vi "Create Data Frame FCS.vi"(0 "Data":u8=128, 1 "OVS":u8=16, 5 "Num_of_FCS_Bits":u8=4, 7 "Polynomial_Mask":u8=19 format="%.0x", 11 "error in (no error)":errorcluster, 12 "sample rate":dbl=1000.0 format="%#_6p") -> (4 "Digital Waveform Graph_Out":digitalwaveform(graph), 15 "error out":errorcluster)   [LabVIEW 2013]
panel:
  out "Final_DATA_Frame":bool[](array[boolean])
  out "All_Decoding_Steps":bool[][](array[boolean])
  out "FCS_Value":u32
  out "Final_Data_FCS":bool[](array[boolean])
  out "Data_FCS":bool[](array[boolean])
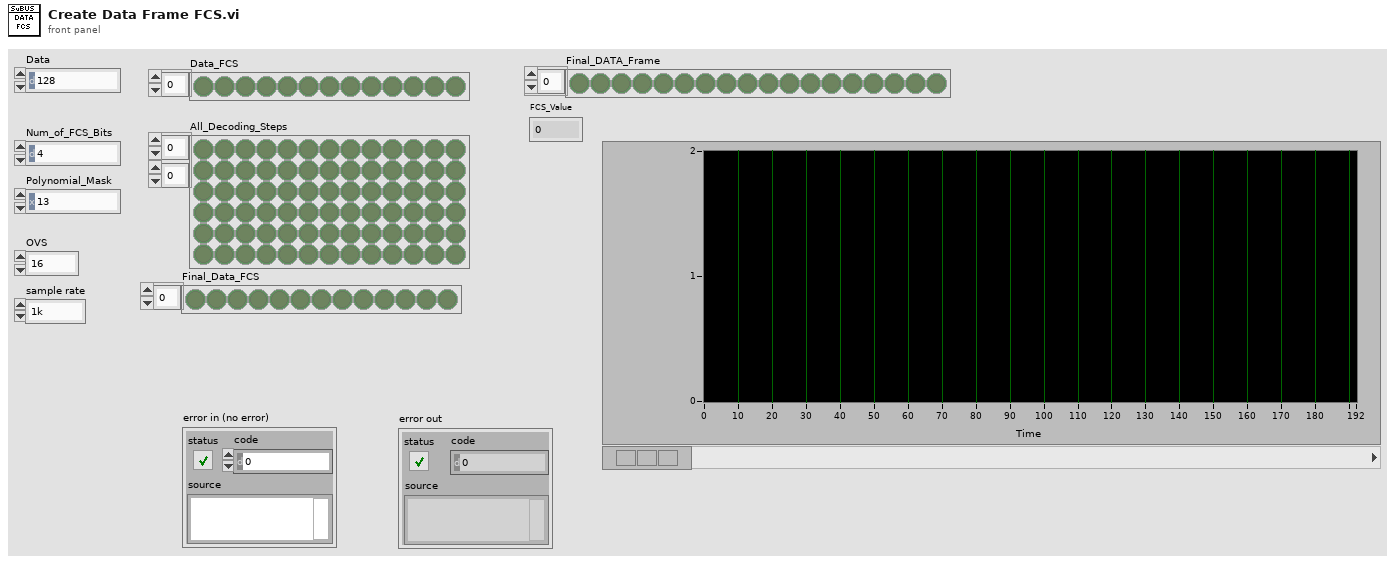
[diagram p1: front panel]
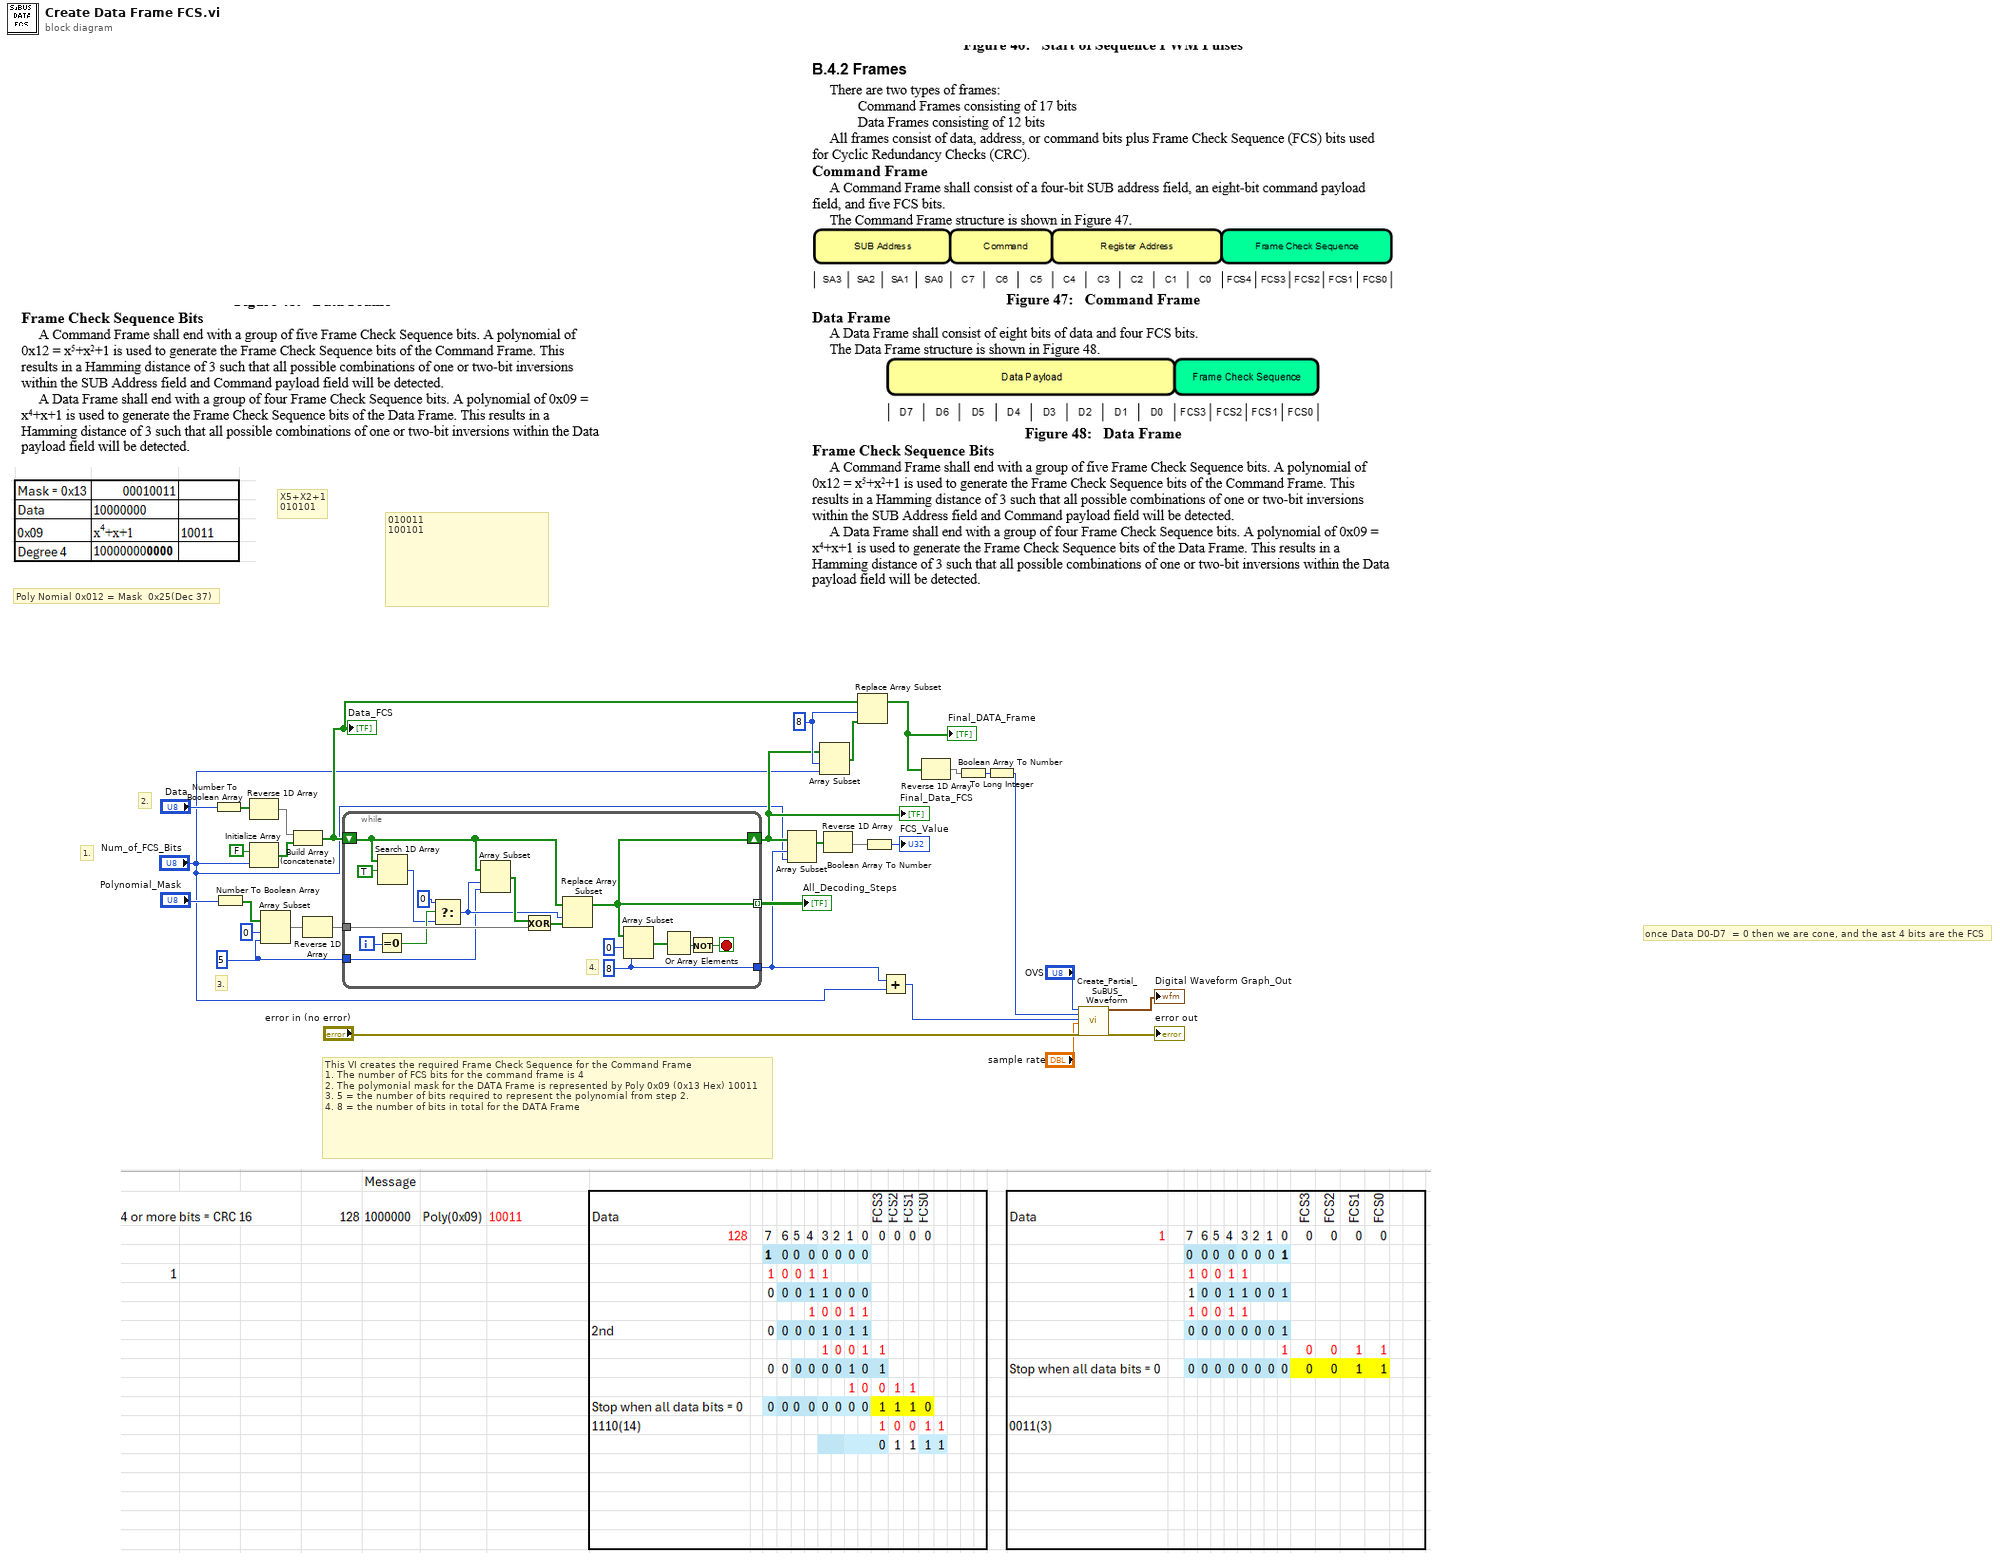
[diagram p0: block diagram]
diagram:
  w6 = 8 ("index")
  w18 = 5 ("length")
  # "3."
  # "2."
  # "1."
  # "This VI creates the required Frame Check Sequence for the Command Frame\n1. The number of FCS bits for the command frame is 4 \n2. The polymonial mask for the DATA Frame is represented by Poly 0x09 (0x13 Hex) 10011\n3. 5 = the number of bits required to represent the polynomial from step 2.\n4. 8 = the number of bits in total for the DATA Frame"
  # "Poly Nomial 0x012 = Mask  0x25(Dec 37)"
  # "010011\n100101"
  # "X5+X2+1\n010101"
  # "once Data D0-D7  = 0 then we are cone, and the ast 4 bits are the FCS"
  n1 = Number To Boolean Array(number="Data") -> (Boolean array=w28:bool[])
  n2 = Number To Boolean Array(number="Polynomial_Mask") -> (Boolean array=w31:bool[])
  n3 = Reverse 1D Array(array=w28) -> (reversed array=w26:bool[])
  n4 = Initialize Array(FALSE ("element"), "Num_of_FCS_Bits") -> (w25:bool[])
  n5 = Array Subset(array=w31, index=0, length=w18) -> (w30:bool[])
  n6 = Build Array (concatenate)(w26, w25) -> (w5:bool[])
  "Data_FCS" <- w5
  n7 = Reverse 1D Array(array=w30) -> (reversed array=w24:bool[])
  n8 = while {
    shift-right: [w34] -> w4
    shift-left: w5 -> [w41]
    tunnel: w24 -> [w48]
    tunnel: [w34] -> w21 mode=indexing
    tunnel: w18 -> [w33]
    tunnel: [w32] -> w10
    i -> [w39]
    stop <- w42 stop-if-true
    w32 = 8 ("length")
    # "4."
    n9 = Equal To 0?(x=w39) -> (x = 0?=w38:bool)
    n10 = Search 1D Array(1D array=w41, element=TRUE) -> (index of element=w37:i32)  [unwired: 1 in]
    n11 = Select(t=0, s=w38, f=w37) -> (s? t:f=w36:i32)
    n12 = Array Subset(array=w41, index=w36, length=w33) -> (w47:bool[])
    n13 = Exclusive Or(1:w48, 2:w47) -> (0:w40:bool[])
    n14 = Replace Array Subset(array=w41, new element=w40, index=w36) -> (w34:bool[])
    n15 = Array Subset(array=w34, index=0, length=w32) -> (w45:bool[])
    n16 = Or Array Elements(Boolean array=w45) -> (logical OR=w44:bool)
    n17 = Not(x=w44) -> (.not. x?=w42:bool)
  }
  "Final_Data_FCS" <- w4
  "All_Decoding_Steps" <- w21
  n18 = Array Subset(array=w4, index=w10, length="Num_of_FCS_Bits") -> (w22:bool[])
  n19 = Array Subset(array=w4, index=w6, length="Num_of_FCS_Bits") -> (w7:bool[])
  n20 = Reverse 1D Array(array=w22) -> (reversed array=w17:bool[])
  n21 = Replace Array Subset(array=w5, new element=w7, index=w6) -> (w1:bool[])
  "Final_DATA_Frame" <- w1
  n22 = Boolean Array To Number(Boolean array=w17) -> (number=→"FCS_Value":u32)
  n23 = Add(x=w10, y="Num_of_FCS_Bits") -> (x+y=w9:i32)
  n24 = Reverse 1D Array(array=w1) -> (reversed array=w2:bool[])
  n25 = Boolean Array To Number(Boolean array=w2) -> (number=w12:u32)
  n26 = To Long Integer(number=w12) -> (32bit integer=w11:i32)
  n27 = call "Create_Partial_SuBUS_Waveform.vi"("OVS"="OVS", "Value"=w11, "Bit_length"=w9, "sample rate"="sample rate", "error in (no error)"="error in (no error)") -> ("Digital Waveform Graph_Out"=→"Digital Waveform Graph_Out":digitalwaveform, "error out"=→"error out":errorcluster)  [unwired: 13 in]
